vi "libssh2_channel_get_exit_status.vi"(8 "error in (no error)":errorcluster, 11 "channel":u64) -> (0 "error out":errorcluster, 3 "return value":i32)   [LabVIEW 2013, in "libssh2.lvlib"]
uses:
  libssh2.lvlib
  libssh2.dll
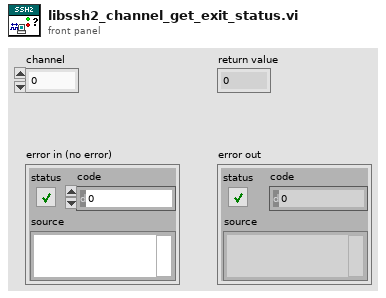
[diagram p1: front panel]
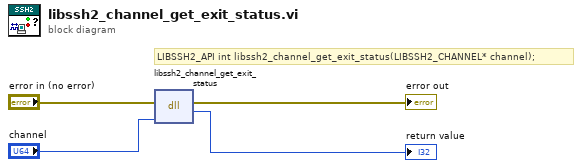
[diagram p0: block diagram]
diagram:
  # "LIBSSH2_API int libssh2_channel_get_exit_status(LIBSSH2_CHANNEL* channel);"
  n1 = dll-call lib="C:/Users/pasca/source/repos/libssh2-labview/libssh2**.*" fn="libssh2_channel_get_exit_status"(error in="error in (no error)", "channel"="channel") -> (error out=→"error out":errorcluster, "return value"=→"return value":i32)  [unwired: 3 in, 1 out]
